vi "Reinitialize.vi"() -> ()   [LabVIEW 2018]
uses:
  <vilib>/nisyscfg/Find Hardware.vi
  <vilib>/nisyscfg/nisyscfg.lvlib
panel:
  in  "error in (no error)":errorcluster
  out "error out":errorcluster
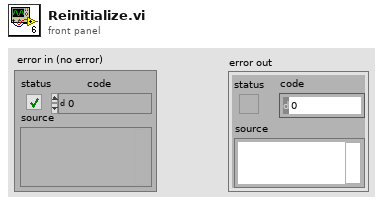
[diagram p1: front panel]
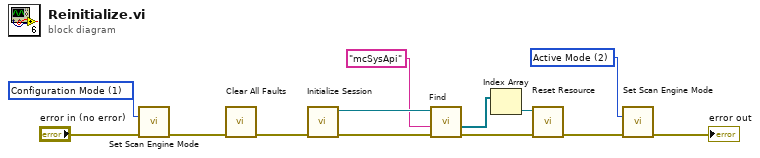
[diagram p0: block diagram]
diagram:
  w4 = 2 items=["Configuration Mode"=1, "Active Mode"=2] ("mode (Active Mode)")
  w6 = 1 items=["Configuration Mode"=1, "Active Mode"=2] ("mode (Active Mode)")
  n1 = call <vilib>:"Set Scan Engine Mode.vi"("mode (Active Mode)"=w6, "error in (no error)"="error in (no error)") -> ("error out"=w2:errorcluster)  [unwired: 13 in]
  n2 = call <vilib>:"Clear All Faults.vi"("error in (no error)"=w2) -> ("error out"=w11:errorcluster)  [unwired: 10 in]
  n3 = call <vilib>:"Initialize Session.vi"("error in (no error)"=w11) -> ("error out"=w12:errorcluster, "Session out"=w13:refnum<k21>)  [unwired: 9 in]
  n4 = call-poly <vilib>:"Find.vi"("error in (no error)"=w12, "Experts"="mcSysApi" ("experts"), "Session in"=w13) -> ("error out"=w1:errorcluster, "Resources out"=w8:refnum<k20>[])  [unwired: 5 in, 2 out]
  n5 = Index Array(array=w8) -> (element=w9:refnum<k20>)  [unwired: 1 in]
  n6 = call <vilib>:"Reset Resource.vi"("error in (no error)"=w1, "Resource in"=w9) -> ("error out"=w5:errorcluster)  [unwired: 6 in, 3 out]
  n7 = call <vilib>:"Set Scan Engine Mode.vi"("mode (Active Mode)"=w4, "error in (no error)"=w5) -> ("error out"=→"error out":errorcluster)  [unwired: 13 in]
